vi "Read fullScale.vi"(8 "error in (no error)":errorcluster, 11 "Alicat in":refnum<class "Alicat.lvclass">) -> (0 "error out":errorcluster, 2 "fullScale":dbl, 3 "Alicat out":refnum<class "Alicat.lvclass">)   [LabVIEW 2013, in "Alicat.lvlib" / "Alicat.lvclass"]
uses:
  Alicat.lvclass
  Alicat.lvclass/Alicat.ctl
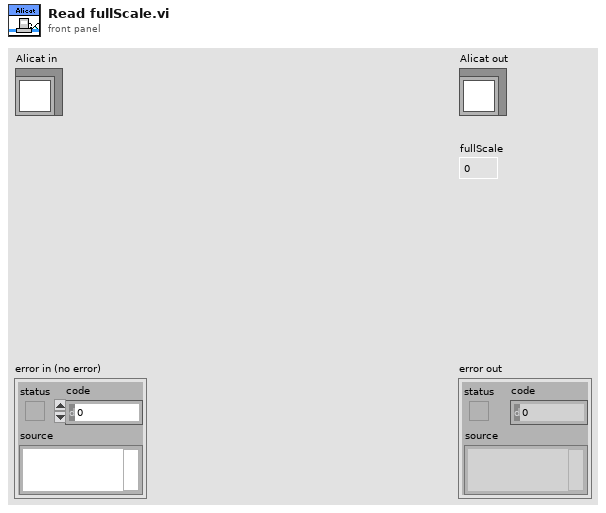
[diagram p1: front panel]
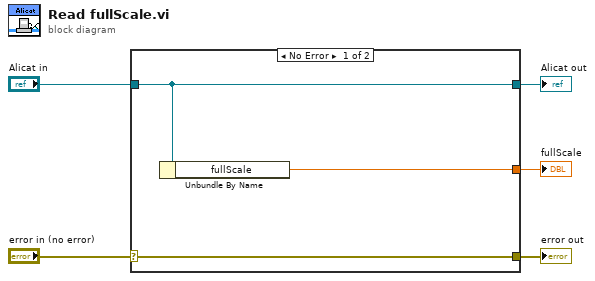
[diagram p0: block diagram]
diagram:
  n1 = case shown="No Error" "error in (no error)" {
    selector: "error in (no error)" -> [w8 w9]
    tunnel: [w8 w9] -> w4
    tunnel: [w7 w10] -> w2
    tunnel: "Alicat in" -> [w7 w10]
    tunnel: [w6 _] -> w1
    frame No Error {
      n2 = Unbundle By Name(w7) -> ("fullScale"=w6:dbl)
    }
    frame Error {
    }
  }
  "error out" <- w4
  "Alicat out" <- w2
  "fullScale" <- w1
